vi "Digital_Read.vi"(8 "error in (no error)":errorcluster, 10 "Pin":u8=4 min=4 max=40, 11 "VISA resource name":refnum<visa-resource-name>) -> (0 "error out":errorcluster, 2 "Valor":bool, 3 "VISA resource name out":refnum<visa-resource-name>)   [LabVIEW 2025]
doc: "Este VI permite enviar una instruccion de lectura digital al pin elegido \nDebe recibir los datos de VISA resource name, Error IN y el pin a leer\nDara como salida VISA resource name, estado logico de lectura y error OUT"
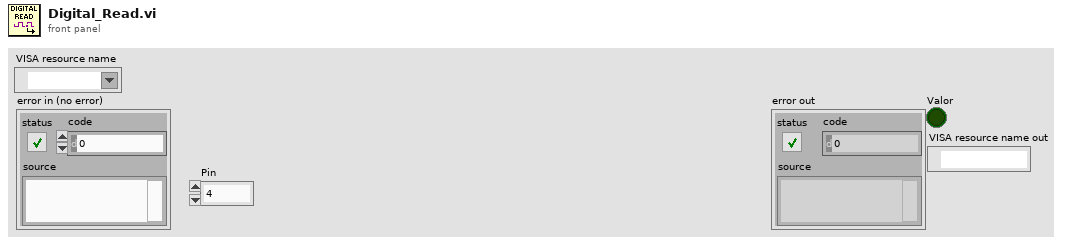
[diagram p1: front panel]
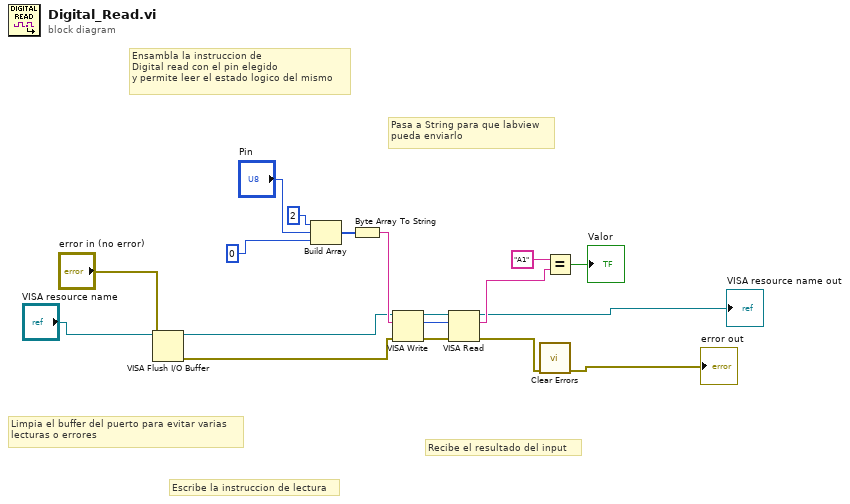
[diagram p0: block diagram]
diagram:
  # "Recibe el resultado del input"
  # "Escribe la instruccion de lectura"
  # "Limpia el buffer del puerto para evitar varias\nlecturas o errores"
  # "Pasa a String para que labview \npueda enviarlo"
  # "Ensambla la instruccion de \nDigital read con el pin elegido\ny permite leer el estado logico del mismo"
  n1 = VISA Flush I/O Buffer(VISA resource name="VISA resource name", error in (no error)="error in (no error)") -> (VISA resource name out=w6:refnum<visa-resource-name>, error out=w5:errorcluster)  [unwired: 1 in]
  n2 = Build Array(u8 2, "Pin", u8 0) -> (w14:u8[])
  n3 = Byte Array To String(unsigned byte array=w14) -> (string=w18:string)
  n4 = VISA Write(VISA resource name=w6, write buffer=w18, error in (no error)=w5) -> (VISA resource name out=w16:refnum<visa-resource-name>, return count=w12:u32, error out=w17:errorcluster)
  n5 = VISA Read(VISA resource name=w16, byte count=w12, error in (no error)=w17) -> (VISA resource name out=→"VISA resource name out":refnum<visa-resource-name>, read buffer=w10:string, error out=w2:errorcluster)  [unwired: 1 out]
  n6 = call <vilib>:"Clear Errors.vi"("error in (no error)"=w2) -> ("error out"=→"error out":errorcluster)  [unwired: 5 in, 1 out]
  n7 = Equal?(x="A1", y=w10) -> (x = y?=→"Valor":bool)
